vi "IMAQ FPGA Image Transfer from Target U16.vi"(6 "Image Transfer Size Alignment":u32(ring)=1 items=["1 Pixel"=1, "8 Pixels"=8], 7 "Read Timeout (ms)":i32=5000, 8 "error in (no error)":errorcluster, 9 "DMA FIFO Reference In":refnum<k20>, 10 "Maximum Pixels per Read":i32=-1, 11 "Image":T1) -> (0 "error out":errorcluster, 1 "DMA FIFO Reference Out":refnum<k20>, 3 "Image Out":T1)   [LabVIEW 2017, in "NI_VDM_FPGA_Basics.lvlib"]
doc: "Transfers an image from the target FPGA to the host processor via DMA FIFO."
uses:
  <vilib>/visionFPGA/NI_VDM_FPGA_Basics.lvlib
  <vilib>/vision/Image Controls.llb/IMAQ Image.ctl
  <vilib>/rvi/errors/niLvFpgaAdjustHostInterfaceError.vi
  <vilib>/rvi/interface/nirviMethod/nirviMethod.xnode
  <vilib>/rvi/errors/niLvFpgaMergeErrorWithErrorCode.vi
  <vilib>/vision/EDVR.llb/IMAQ ImageToEDVR 2D U16.vi
  nivissvc.dll
  <vilib>/FPGAPlugInAG/Dynamic/niLvFpga_AcquireReadRegionFifo_Dynamic.vi
  <vilib>/FPGAPlugInAG/Dynamic/niLvFpga_ReadFifo_Dynamic.vi
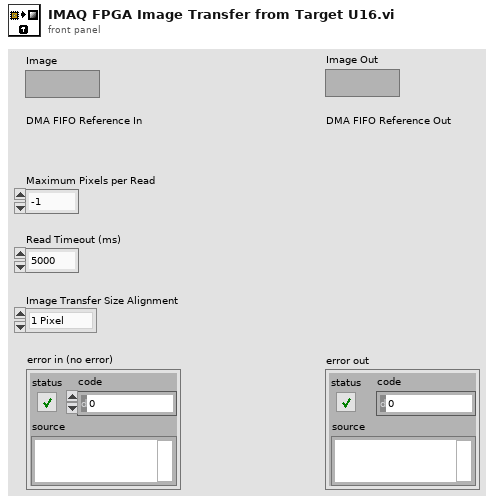
[diagram p1: front panel]
types:
  T1 = typedef "IMAQ Image.ctl" = refnum<image>
  T2 = typedef "Image Type" = u32
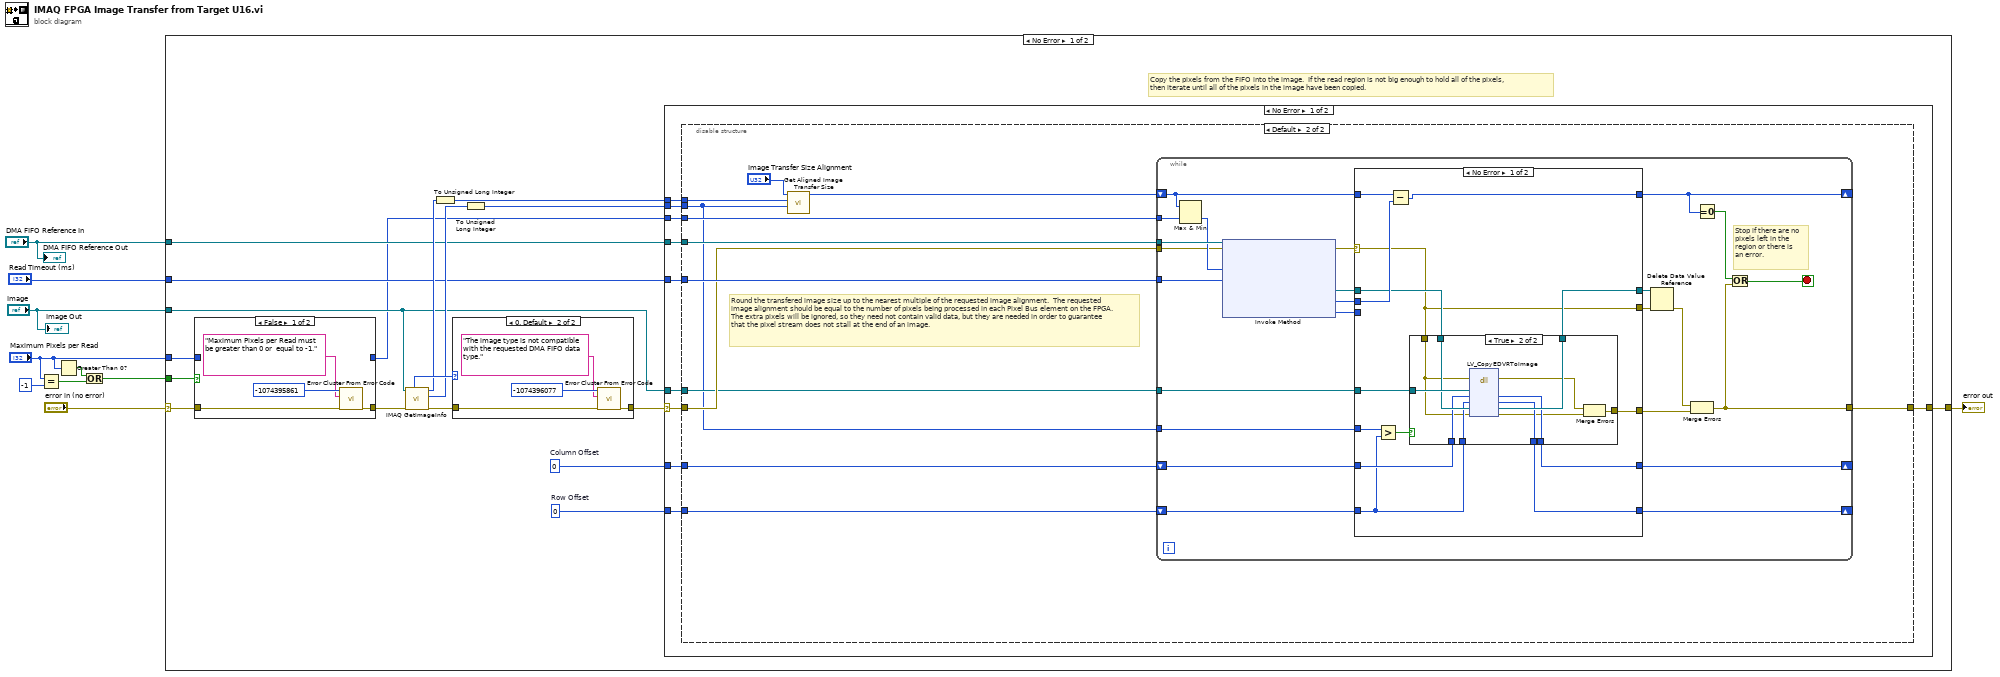
[diagram p0: block diagram]
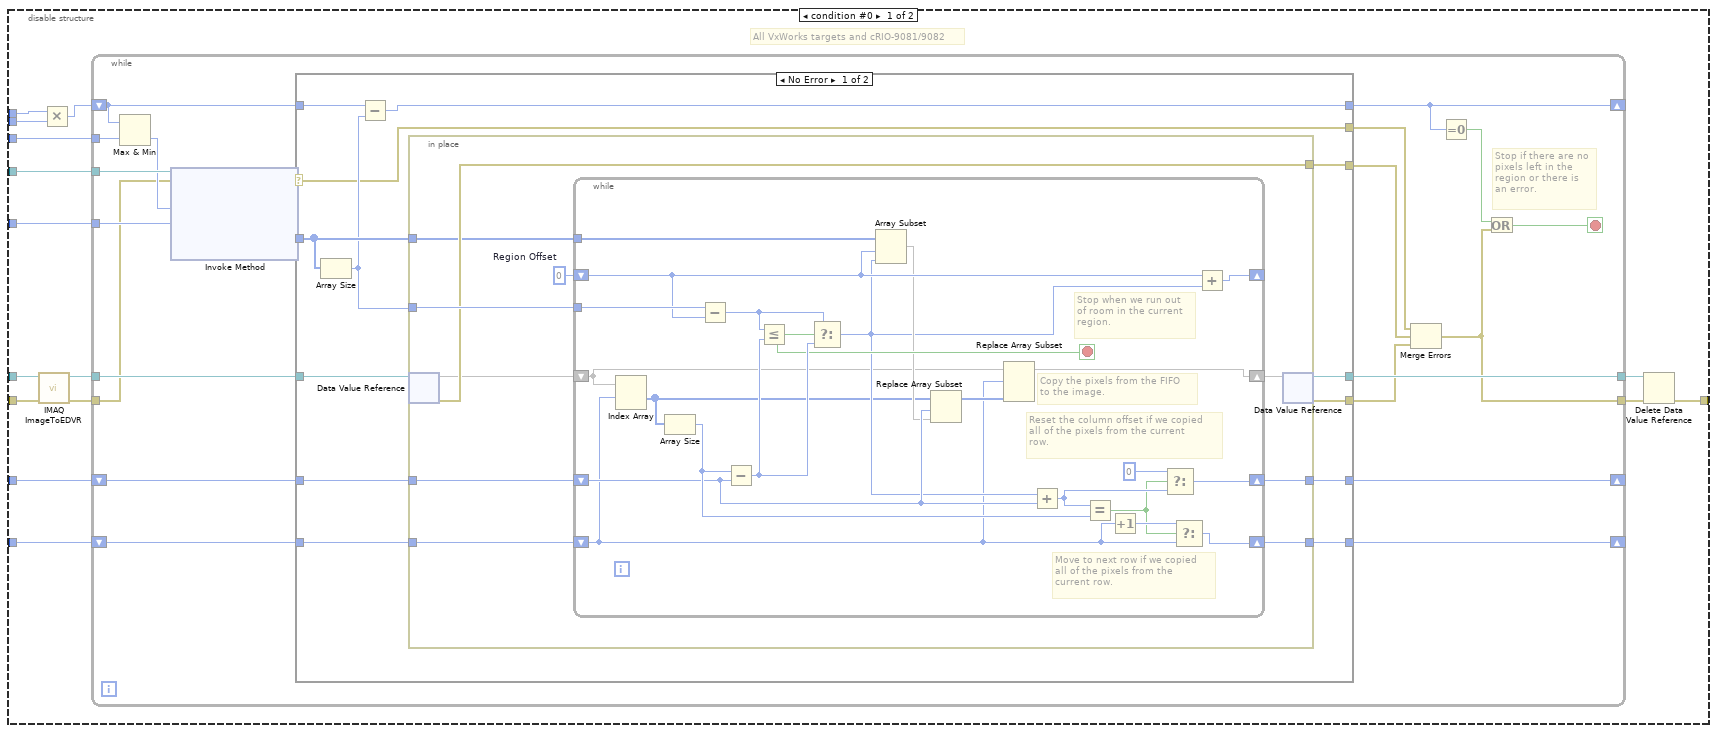
[diagram p2: hidden frame]
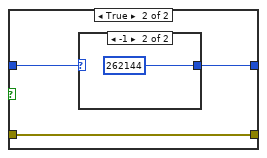
[diagram p7: hidden frame]
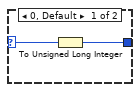
[diagram p8: hidden frame]
diagram:
  n1 = Equal?(x="Maximum Pixels per Read", y=-1) -> (x = y?=w6:bool)
  n2 = Greater Than 0?(x="Maximum Pixels per Read") -> (x > 0?=w7:bool)
  n3 = Or(x=w7, y=w6) -> (x .or. y?=w4:bool)
  n4 = case shown="No Error" "error in (no error)" {
    selector: "error in (no error)" -> [w23 w211]
    tunnel: "Read Timeout (ms)" -> [w15 _]
    tunnel: "DMA FIFO Reference In" -> [w14 _]
    tunnel: "Maximum Pixels per Read" -> [w25 _]
    tunnel: w4 -> [w24 _]
    tunnel: "Image" -> [w16 _]
    tunnel: [w21 w211] -> w2
    frame No Error {
      w20 = u32 0  # Row Offset
      w19 = u32 0  # Column Offset
      # "Copy the pixels from the FIFO into the image.  If the read region is not big enough to hold all of the pixels,\nthen iterate until all of the pixels in the image have been copied."
      n5 = case shown="False" w24 {
        tunnel: w23 -> [w197 w202]
        tunnel: [w196 w202] -> w26
        tunnel: w25 -> [_ w201]
        tunnel: [_ w200] -> w13
        frame False {
          n6 = call <vilib>:"Error Cluster From Error Code.vi"("error in (no error)"=w197, "error message (\"\")"="Maximum Pixels per Read must be greater than 0 or  equal to -1." ("error message (\"\")"), "error code (0)"=-1074395861) -> ("error out"=w196:errorcluster)  [unwired: 6 in]
        }
        frame True {
          n7 = case shown="-1" w201 {
            selector: w201 -> [w204 _]
            tunnel: [w203 u32 262144 ("Maximum Pixels per Write")] -> w200
            frame 0, Default {
              n8 = To Unsigned Long Integer(number=w204) -> (unsigned 32bit integer=w203:u32)
            }
            frame -1 {
            }
          }
        }
      }
      n9 = call "IMAQ GetImageInfo"("error in (no error)"=w26, "Image"=w16) -> ("error out"=w27:errorcluster, "Y Resolution"=w18:i32, "X Resolution"=w22:i32, "Image Type"=w28:T2)  [unwired: 2 in, 4 out]
      n10 = To Unsigned Long Integer(number=w22) -> (unsigned 32bit integer=w12:u32)
      n11 = case shown="0, Default" w28 {
        tunnel: w27 -> [w206 w208]
        tunnel: [w206 w207] -> w17
        frame 1, 7 {
          # "Allowed types are:\nGrayscale (I16)\nGrayscale (U16)"
        }
        frame 0, Default {
          n12 = call <vilib>:"Error Cluster From Error Code.vi"("error in (no error)"=w208, "error message (\"\")"="The image type is not compatible with the requested DMA FIFO data type." ("error message (\"\")"), "error code (0)"=-1074396077) -> ("error out"=w207:errorcluster)  [unwired: 6 in]
        }
      }
      n13 = To Unsigned Long Integer(number=w18) -> (unsigned 32bit integer=w11:u32)
      n14 = case shown="No Error" w17 {
        selector: w17 -> [w37 w195]
        tunnel: w19 -> [w36 _]
        tunnel: w20 -> [w35 _]
        tunnel: w14 -> [w33 _]
        tunnel: [w31 w195] -> w21
        tunnel: w13 -> [w32 _]
        tunnel: w15 -> [w34 _]
        tunnel: w16 -> [w38 _]
        tunnel: w12 -> [w30 _]
        tunnel: w11 -> [w29 _]
        frame No Error {
          n15 = disable-structure shown="Default" {
            disable-tunnel: w36 -> [w53 w136]
            disable-tunnel: w35 -> [w52 w135]
            disable-tunnel: w33 -> [w51 w134]
            disable-tunnel: [w42 w133] -> w31
            disable-tunnel: w32 -> [w50 w132]
            disable-tunnel: w34 -> [w49 w131]
            disable-tunnel: w38 -> [w48 w129]
            disable-tunnel: w37 -> [w46 w130]
            disable-tunnel: w30 -> [w39 w126]
            disable-tunnel: w29 -> [w40 w125]
            frame condition #0 {
              # "All VxWorks targets and cRIO-9081/9082"
              n16 = call-poly <vilib>:"IMAQ ImageToEDVR.vi"("error out"=w46, "Image"=w48) -> ("error out"=w45:errorcluster, "EDVR 2D U16"=w47:refnum<data-value>)  [unwired: 7 in, 1 out]
              n17 = Multiply(x=w39, y=w40) -> (x*y=w41:u32)
              n18 = while {
                shift-right: [w65] -> _
                shift-left: w41 -> [w61]
                shift-right: [w70] -> _
                shift-left: w53 -> [w72]
                shift-right: [w73] -> _
                shift-left: w52 -> [w71]
                tunnel: w51 -> [w69]
                tunnel: [w67] -> w44
                tunnel: [w63] -> w43
                tunnel: w50 -> [w59]
                tunnel: w49 -> [w58]
                tunnel: w47 -> [w55]
                tunnel: w45 -> [w54]
                stop <- w64 stop-if-true
                # "Stop if there are no\npixels left in the \nregion or there is\nan error."
                n19 = Max & Min(x=w61, y=w59) -> (min(x,y)=w60:u32)  [unwired: 1 out]
                n20 = xnode "Invoke Method"("FPGA VI Reference In"=w69, "error in"=w54, "Number of Elements"=w60, "Timeout (ms)"=w58) -> ("error out"=w68:errorcluster, "Data"=w74:u16[])  [unwired: 2 out]
                n21 = case shown="No Error" w68 {
                  selector: w68 -> [w75 w120]
                  tunnel: w61 -> [w87 w123]
                  tunnel: [w86 w123] -> w65
                  tunnel: w55 -> [w85 w124]
                  tunnel: w74 -> [w77 _]
                  tunnel: [w84 w121] -> w73
                  tunnel: w72 -> [w83 w122]
                  tunnel: w71 -> [w82 w121]
                  tunnel: [w81 w122] -> w70
                  tunnel: [w80 w124] -> w67
                  tunnel: [w75 w120] -> w57
                  tunnel: [w79 _] -> w56
                  tunnel: [w78 _] -> w66
                  frame No Error {
                    n22 = Array Size(array=w77) -> (size(s)=w76:i32)
                    n23 = Subtract(x=w87, y=w76) -> (x-y=w86:u32)
                    n24 = in-place {
                      in-place-border: w76 -> [w95]
                      in-place-border: [w97] -> w84
                      in-place-border: w83 -> [w94]
                      in-place-border: w82 -> [w90]
                      in-place-border: [w93] -> w81
                      in-place-border: [w92] -> w78
                      in-place-border: w77 -> [w88]
                      w96 = u32 0  # Region Offset
                      n25 = in-place-dvr #1(w85) -> (w91:u16[][], w92:errorcluster)
                      n26 = while {
                        shift-right: [w117] -> _
                        shift-left: w96 -> [w116]
                        tunnel: w88 -> [w106]
                        tunnel: w95 -> [w119]
                        shift-right: [w111] -> w93
                        shift-left: w94 -> [w107]
                        shift-right: [w98] -> w89
                        shift-left: w91 -> [w101]
                        shift-right: [w109] -> w97
                        shift-left: w90 -> [w99]
                        stop <- w108 stop-if-true
                        # "Stop when we run out\nof room in the current\nregion."
                        # "Copy the pixels from the FIFO\nto the image."
                        # "Reset the column offset if we copied\nall of the pixels from the current\nrow."
                        # "Move to next row if we copied\nall of the pixels from the\ncurrent row."
                        n27 = Index Array(array=w101, index (row)=w99) -> (element=w102:u16[])  [unwired: 1 in]
                        n28 = Array Size(array=w102) -> (size(s)=w115:i32)
                        n29 = Subtract(x=w119, y=w116) -> (x-y=w118:u32)
                        n30 = Subtract(x=w115, y=w107) -> (x-y=w114:u32)
                        n31 = Less Or Equal?(x=w118, y=w114) -> (x <= y?=w108:bool)
                        n32 = Select(t=w118, s=w108, f=w114) -> (s? t:f=w104:u32)
                        n33 = Array Subset(array=w106, index=w116, length=w104) -> (w105:u16[])
                        n34 = Replace Array Subset(array=w102, new element=w105, index=w107) -> (w100:u16[])
                        n35 = Replace Array Subset(array=w101, new element=w100, index (row)=w99) -> (w98:u16[][])  [unwired: 1 in]
                        n36 = Add(x=w104, y=w107) -> (x+y=w112:u32)
                        n37 = Equal?(x=w112, y=w115) -> (x = y?=w103:bool)
                        n38 = Increment(x=w99) -> (x+1=w110:u32)
                        n39 = Select(t=u32 0 ("Elements In Region"), s=w103, f=w112) -> (s? t:f=w111:u32)
                        n40 = Select(t=w110, s=w103, f=w99) -> (s? t:f=w109:u32)
                        n41 = Add(x=w116, y=w104) -> (x+y=w117:u32)
                      }
                      n42 = in-place-dvr #1(w89) -> (w80:refnum<data-value>, w79:errorcluster)
                    }
                  }
                  frame Error {
                  }
                }
                n43 = Merge Errors(w57, w66, w56) -> (w63:errorcluster)
                n44 = Equal To 0?(x=w65) -> (x = 0?=w62:bool)
                n45 = Or(x=w62, y=w63) -> (x .or. y?=w64:bool)
              }
              n46 = Delete Data Value Reference(data value reference=w44, error in=w43) -> (error out=w42:errorcluster)  [unwired: 1 out]
            }
            frame condition #1 (active) {
              # "Round the transfered image size up to the nearest multiple of the requested image alignment.  The requested image alignment should be equal to the number of pixels being processed in each Pixel Bus element on the FPGA.  The extra pixels will be ignored, so they need not contain valid data, but they are needed in order to guarantee that the pixel stream does not stall at the end of an image."
              n47 = call <vilib>:"Get Aligned Image Transfer Size.vi"("Y Resolution"=w125, "X Resolution"=w126, "Image Transfer Size Alignment"="Image Transfer Size Alignment") -> ("Aligned Image Transfer Size"=w127:u64)  [unwired: 8 in]
              n48 = while {
                shift-right: [w151] -> _
                shift-left: w127 -> [w148]
                shift-right: [w155] -> _
                shift-left: w136 -> [w157]
                shift-right: [w158] -> _
                shift-left: w135 -> [w156]
                tunnel: w134 -> [w154]
                tunnel: [w138] -> w133
                tunnel: w132 -> [w145]
                tunnel: w131 -> [w144]
                tunnel: w130 -> [w143]
                tunnel: w129 -> [w142]
                tunnel: w125 -> [w137]
                stop <- w150 stop-if-true
                # "Stop if there are no\npixels left in the \nregion or there is\nan error."
                n49 = Max & Min(x=w148, y=w145) -> (min(x,y)=w147:u64)  [unwired: 1 out]
                n50 = xnode "Invoke Method"("FPGA VI Reference In"=w154, "error in"=w143, "Number of Elements"=w147, "Timeout (ms)"=w144) -> ("error out"=w153:errorcluster, "Read Region Reference"=w160:refnum<data-value>, "Elements In Region"=w159:u32, "Elements Remaining"=w146:u32)  [unwired: 1 out]
                n51 = case shown="No Error" w153 {
                  selector: w153 -> [w164 w190]
                  tunnel: w148 -> [w174 w194]
                  tunnel: [w173 w194] -> w151
                  tunnel: w160 -> [w169 w191]
                  tunnel: w159 -> [w170 _]
                  tunnel: [w166 w192] -> w158
                  tunnel: w157 -> [w168 w193]
                  tunnel: w156 -> [w162 w192]
                  tunnel: [w167 w193] -> w155
                  tunnel: [w171 w191] -> w152
                  tunnel: [w164 w190] -> w141
                  tunnel: w146 -> [_ _]
                  tunnel: w142 -> [w172 _]
                  tunnel: [w165 w190] -> w140
                  tunnel: w137 -> [w161 _]
                  frame No Error {
                    n52 = Greater?(x=w161, y=w162) -> (0:w163:bool)
                    n53 = Subtract(x=w174, y=w170) -> (x-y=w173:u64)
                    n54 = case shown="True" w163 {
                      tunnel: w172 -> [_ w189]
                      tunnel: [w177 w188] -> w171
                      tunnel: w169 -> [w177 w187]
                      tunnel: w168 -> [w175 w186]
                      tunnel: w162 -> [w176 w185]
                      tunnel: [w175 w184] -> w167
                      tunnel: [w176 w183] -> w166
                      tunnel: [w178 w180] -> w165
                      tunnel: w164 -> [w178 w179]
                      frame False {
                      }
                      frame True {
                        n55 = dll-call lib="nivissvc.*" fn="LV_CopyEDVRToImage"(error in=w179, "image"=w189, "xImageOffset"=w186, "yImageOffset"=w185, "EDVR"=w187, "error"=w179) -> (error out=w181:errorcluster, "xImageOffset"=w184:u32, "yImageOffset"=w183:u32, "EDVR"=w188:refnum<data-value>, "error"=w182:errorcluster)  [unwired: 4 in, 1 out]
                        n56 = Merge Errors(w181, w182) -> (w180:errorcluster)
                      }
                    }
                  }
                  frame Error {
                  }
                }
                n57 = Delete Data Value Reference(data value reference=w152, error in=w141) -> (error out=w139:errorcluster)  [unwired: 1 out]
                n58 = Merge Errors(w139, w140) -> (w138:errorcluster)
                n59 = Equal To 0?(x=w151) -> (x = 0?=w149:bool)
                n60 = Or(x=w149, y=w138) -> (x .or. y?=w150:bool)
              }
            }
          }
        }
        frame Error {
        }
      }
    }
    frame Error {
    }
  }
  "error out" <- w2
  "Image Out" <- "Image"
  "DMA FIFO Reference Out" <- "DMA FIFO Reference In"
